vi "Create Grid.vi"(11 "String":string) -> (3 "Array":string[][](array[string]))   [LabVIEW 2021]
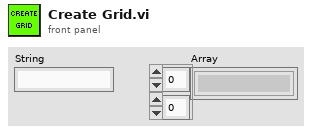
[diagram p1: front panel]
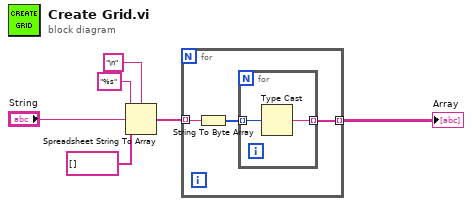
[diagram p0: block diagram]
diagram:
  n1 = Spreadsheet String To Array(delimiter (Tab)="\n", format string="%s", spreadsheet string="String", array type (2D Dbl)=string[] []) -> (array=w5:string[])
  n2 = for {
    tunnel: w5 -> [w9] mode=indexing
    tunnel: [w7] -> w6 mode=indexing
    n3 = String To Byte Array(string=w9) -> (unsigned byte array=w8:u8[])
    n4 = for {
      tunnel: w8 -> [w11] mode=indexing
      tunnel: [w10] -> w7 mode=indexing
      n5 = Type Cast(x=w11) -> (*(type *) &x=w10:string)  [unwired: 1 in]
    }
  }
  "Array" <- w6
